vi "Test Item Indent Correct for Method.vi"(8 "error in (no error)":errorcluster, 11 "Result Model Tests in":refnum<class "Result Model Test Enumeration.lvclass">) -> (0 "error out":errorcluster, 3 "Result Model Tests out":refnum<class "Result Model Test Enumeration.lvclass">)   [LabVIEW 2020, in "Result Model Test Enumeration.lvclass"]
uses:
  Result Model Test Enumeration.lvclass
  source/User Interface/Result Model/Result Model.lvclass
  206db1ee-aa99-40b9-8881-171f2a77c34b.vi
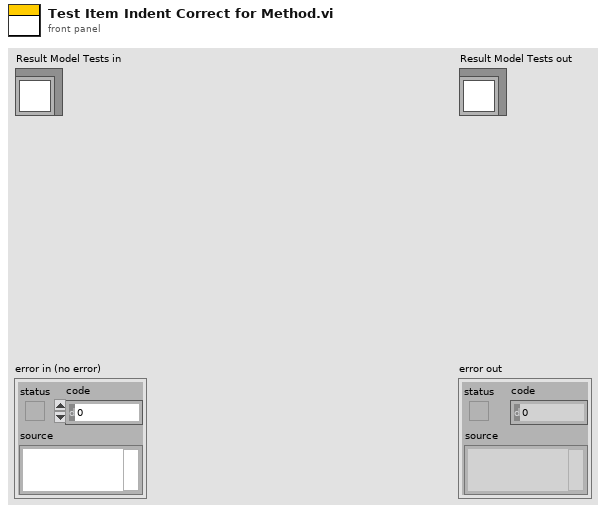
[diagram p1: front panel]
types:
  T1 = cluster{"Left Cell String":string, "Child Text":string[], "Child Tag":string, "Item Indent":i32, "Child Only?":bool, "Glyph Index":i32}[]
  T2 = cluster{"Left Cell String":string, "Child Text":string[], "Child Tag":string, "Item Indent":i32, "Child Only?":bool, "Glyph Index":i32}
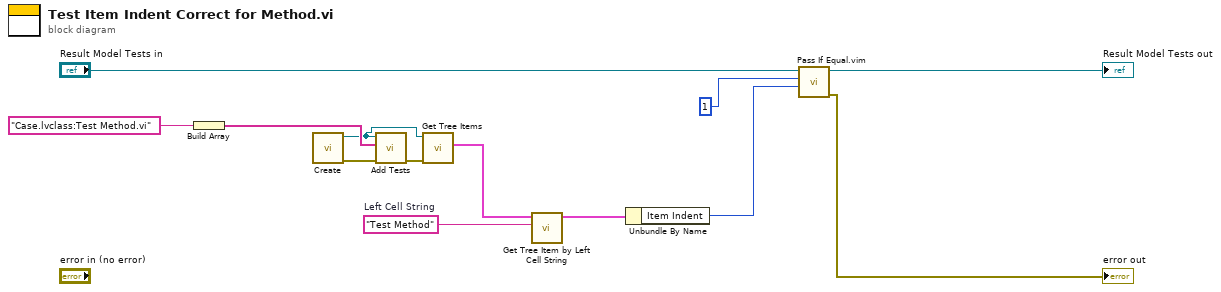
[diagram p0: block diagram]
diagram:
  w5 = "Test Method"  # Left Cell String
  n1 = Build Array("Case.lvclass:Test Method.vi" ("String")) -> (w8:string[])
  n2 = call "Create.vi"() -> ("error out"=w3:errorcluster, "Result Model out"=w1:refnum<class "Result Model.lvclass">)  [unwired: 10 in]
  n3 = call "Add Tests.vi"("error in (no error)"=w3, "Tests"=w8, "Result Model by Reference In"=w1) -> ("error out"=w2:errorcluster)  [unwired: 8 in]
  n4 = call "Get Tree Items.vi"("error in (no error)"=w2, "Result Model by Reference In"=w1) -> ("Tree Items"=w12:T1)  [unwired: 8 in, 1 out]
  n5 = call "Get Tree Item by Left Cell String.vi"("Left Cell String"=w5, "Tree Items"=w12) -> ("Item"=w10:T2)  [unwired: 9 in]
  n6 = Unbundle By Name(w10) -> ("Item Indent"=w9:i32)
  n7 = call "Pass If Equal.vim"("Actual"=w9, "Expected"=1 ("Item Indent"), "LUnit Test Case In"="Result Model Tests in") -> ("error out"=→"error out":errorcluster, "LUnit Test Case Out"=→"Result Model Tests out":refnum<class "Result Model Test Enumeration.lvclass">)  [unwired: 7 in]
